vi "4Pi Focus Lock - 2D Gaussian - Fit -init.vi"(0 "Image In (DBL)":dbl[][](array[numeric]), 9 "width":dbl, 11 "Error In":errorcluster) -> (8 "Best Fit Params":T1, 15 "Error Out":errorcluster)   [LabVIEW 2016]
uses:
  Tools/2D Gaussian Fit/2D Gaussian - Type Defs/2D Gaussian - Best Fit Parameters.ctl
  4Pi Objective Lock - EMBL/4Pi Objective Lock Type Defs/4Pi OBJ Lock-2D Gaussian - Best Fit Parameters.ctl
  <vilib>/gmath/NumericalOptimization/Nonlinear Curve Fit LM bound.vi
  <vilib>/gmath/NI_Gmath.lvlib
panel:
  out "MSE":dbl
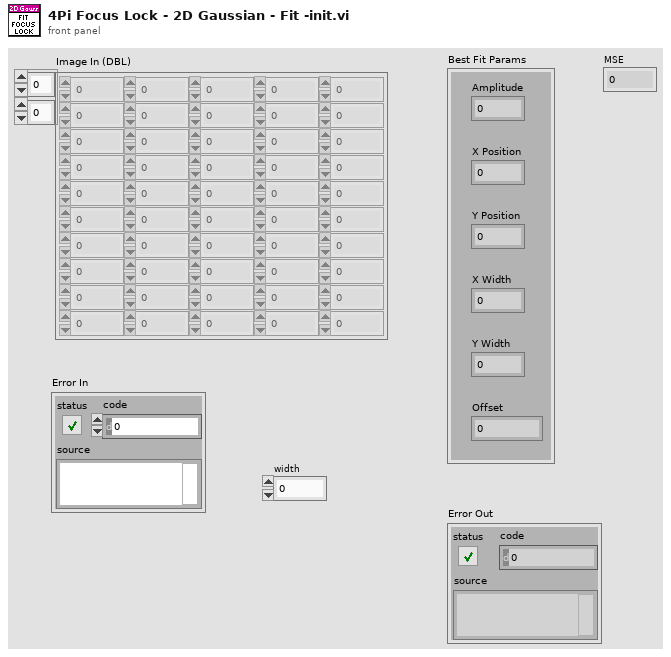
[diagram p1: front panel]
types:
  T1 = typedef "2D Gaussian - Best Fit Parameters.ctl" = cluster{"Amplitude":dbl, "X Position":dbl, "Y Position":dbl, "X Width":dbl, "Y Width":dbl, "Offset":dbl}
  T2 = typedef "4Pi OBJ Lock-2D Gaussian - Best Fit Parameters.ctl" = cluster{"Amplitude":dbl, "X Position":dbl, "Y Position":dbl, "X Width":dbl, "Y Width":dbl, "Offset":dbl}
  T3 = cluster{"parameter minimum":dbl[], "parameter maximum":dbl[]}
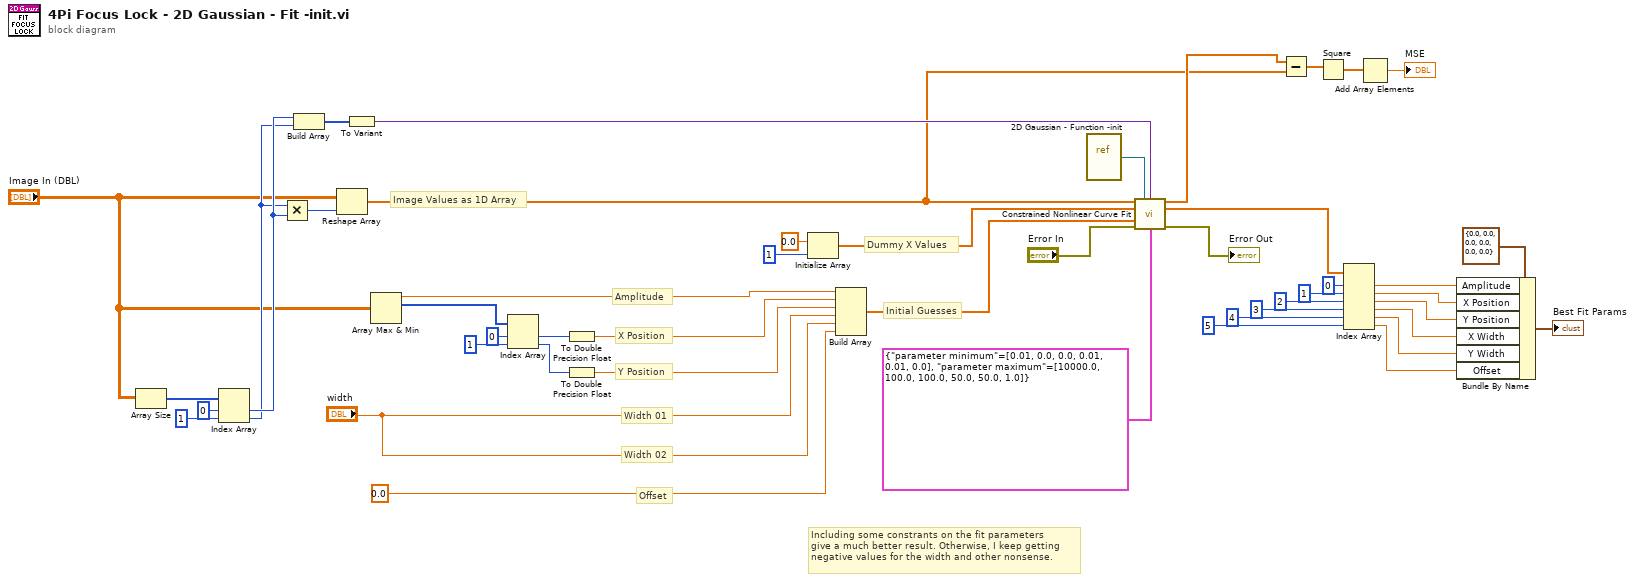
[diagram p0: block diagram]
diagram:
  # "Including some constrants on the fit parameters\ngive a much better result. Otherwise, I keep getting\nnegative values for the width and other nonsense."
  # "Dummy X Values"
  # "Image Values as 1D Array"
  # "Initial Guesses"
  # "Width 02"
  # "Width 01"
  # "Y Position"
  # "X Position"
  # "Offset"
  # "Amplitude"
  n1 = Array Size(array="Image In (DBL)") -> (size(s)=w37:i32[])
  n2 = Index Array(array=w37, index #1=0 ("index"), index #2=1 ("index")) -> (element #1=w31:i32, element #2=w30:i32)
  n3 = Multiply(x=w30, y=w31) -> (x*y=w36:i32)
  n4 = Build Array(w31, w30) -> (w29:i32[])
  n5 = Reshape Array("Image In (DBL)", w36) -> (w4:dbl[])
  n6 = To Variant(anything=w29) -> (Variant=w28:variant)
  n7 = Array Max & Min(array="Image In (DBL)") -> (max value=w8:dbl, max index (indices)=w46:i32[])  [unwired: 2 out]
  n8 = Index Array(array=w46, index #1=0 ("index"), index #2=1 ("index")) -> (element #1=w43:i32, element #2=w41:i32)
  n9 = To Double Precision Float(number=w43) -> (double precision float=w42:dbl)
  n10 = To Double Precision Float(number=w41) -> (double precision float=w40:dbl)
  n11 = Initialize Array(0.0 ("element"), 1 ("dimension size")) -> (w34:dbl[])
  n12 = Build Array(w8, w42, w40, "width", "width", 0.0 ("element")) -> (w33:dbl[])
  n13 = vi-ref "2D Gaussian - Function -init.vi"() -> (w47:refnum<vi>)
  n14 = call-poly <vilib>:"Constrained Nonlinear Curve Fit.vi"("Y"=w4, "f(x,a)"=w47, "data"=w28, "X"=w34, "initial parameters"=w33, "error in (no error)"="Error In", "parameter bounds"=T3 {"parameter minimum"=[0.01, 0.0, 0.0, 0.01, 0.01, 0.0], "parameter maximum"=[10000.0, 100.0, 100.0, 50.0, 50.0, 1.0]}) -> ("best nonlinear fit"=w5:dbl[], "best fit parameters"=w26:dbl[], "error out"=→"Error Out":errorcluster)  [unwired: 3 in, 3 out]
  n15 = Subtract(x=w5, y=w4) -> (x-y=w3:dbl[])
  n16 = Square(x=w3) -> (x^2=w2:dbl[])
  n17 = Index Array(array=w26, index #1=0 ("index"), index #2=1 ("index"), index #3=2 ("index"), index #4=3 ("index"), index #5=4 ("index"), index #6=5 ("index")) -> (element #1=w25:dbl, element #2=w24:dbl, element #3=w23:dbl, element #4=w22:dbl, element #5=w21:dbl, element #6=w20:dbl)
  n18 = Add Array Elements(numeric array=w2) -> (sum=→"MSE":dbl)
  n19 = Bundle By Name(cluster=T2 {"Amplitude"=0.0, "X Position"=0.0, "Y Position"=0.0, "X Width"=0.0, "Y Width"=0.0, "Offset"=0.0} ("Best Fit Parameters"), "Amplitude"=w25, "X Position"=w24, "Y Position"=w23, "X Width"=w22, "Y Width"=w21, "Offset"=w20) -> (→"Best Fit Params":T2)
